vi "File Stop.vi"(8 "Error In":errorcluster) -> (0 "Error Out":errorcluster)   [LabVIEW 2017, in "Toolkit.lvlib"]
doc: "Stop writing logging statements and closes the default logging file."
uses:
  Toolkit.lvlib
  Support VIs/Control Action.ctl
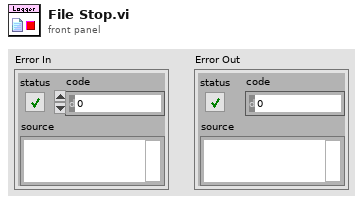
[diagram p1: front panel]
types:
  T1 = typedef "Toolkit.lvlib/Control Action.ctl" = enum16{"Initialize", "Get", "Set", "Shutdown"}
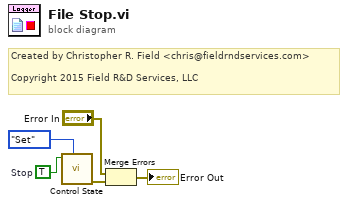
[diagram p0: block diagram]
diagram:
  w4 = TRUE  # Stop
  # "Created by Christopher R. Field <chris@fieldrndservices.com>\n\nCopyright 2015 Field R&D Services, LLC"
  n1 = call "Control State.vi"("Action"=Control_Action."Set", "Set Value"=w4) -> ("Error Out"=w2:errorcluster)  [unwired: 8 in, 1 out]
  n2 = Merge Errors("Error In", w2) -> (→"Error Out":errorcluster)
